vi "ADC_write_read.vi"(8 "Sync_cnt":bool=TRUE, 11 "ADC  in":bool[](array[boolean])) -> (1 "ADC FIFO SYNC":u16=65532 format="%016b", 2 "ADC in":u32[](array[numeric]), 3 "ADC out":u32[](array[numeric]))   [LabVIEW 2015]
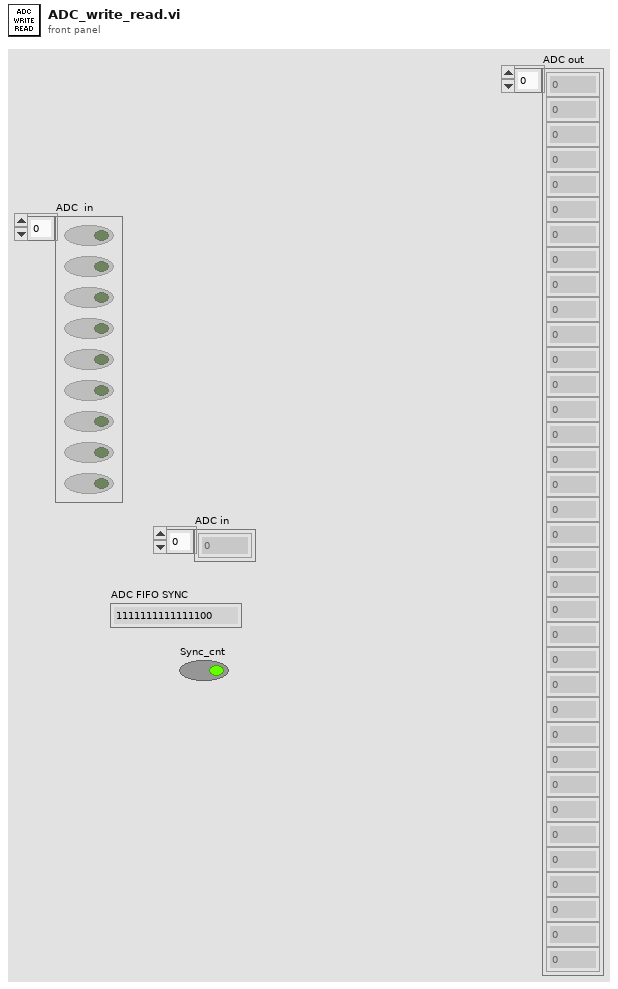
[diagram p1: front panel]
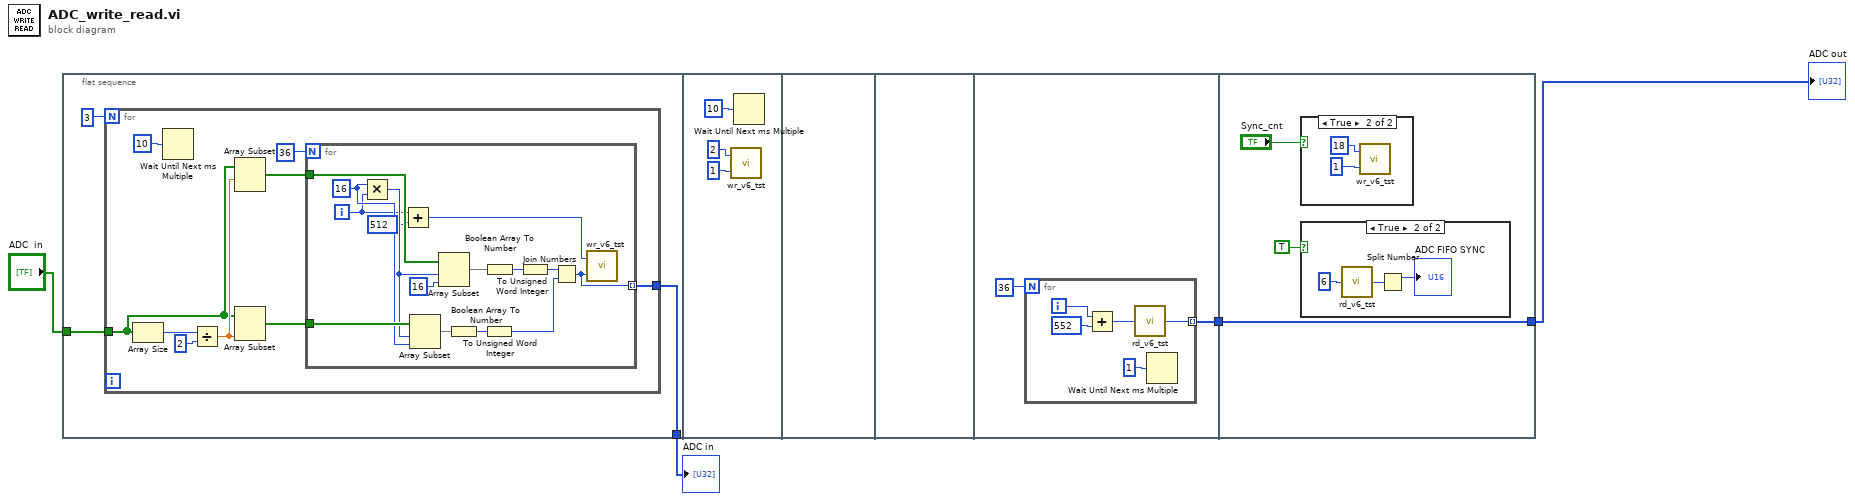
[diagram p0: block diagram]
diagram:
  n1 = flat-sequence {
    tunnel: "ADC  in" -> [w7]
    tunnel: [w6] -> w4
    tunnel: [w35] -> w2
    tunnel: [w44] -> w1
    tunnel: w2 -> [w44]
    frame #0 {
      n2 = for {
        N: 3 -> [_]
        tunnel: w7 -> [w10]
        tunnel: [w9] -> w6
        n3 = Array Size(array=w10) -> (size(s)=w11:i32)
        n4 = Wait Until Next ms Multiple(millisecond multiple=u32 10) -> ()  [unwired: 1 out]
        n5 = Divide(x=w11, y=2) -> (x/y=w16:dbl)
        n6 = Array Subset(array=w10, index=w16) -> (w14:bool[])  [unwired: 1 in]
        n7 = Array Subset(array=w10, length=w16) -> (w13:bool[])  [unwired: 1 in]
        n8 = for {
          N: 36 -> [_]
          tunnel: w13 -> [w31]
          tunnel: w14 -> [w29]
          tunnel: [w19] -> w9 mode=indexing
          i -> [w20]
          w30 = 16 ("length")
          n9 = Multiply(x=w30, y=w20) -> (x*y=w27:i32)
          n10 = Add(x=w20, y=512) -> (x+y=w18:i32)
          n11 = Array Subset(array=w31, index=w27, length=w30) -> (w23:bool[])
          n12 = Array Subset(array=w29, index=w27, length=16) -> (w24:bool[])
          n13 = Boolean Array To Number(Boolean array=w23) -> (number=w25:u32)
          n14 = To Unsigned Word Integer(number=w25) -> (unsigned 16bit integer=w22:u16)
          n15 = Boolean Array To Number(Boolean array=w24) -> (number=w26:u32)
          n16 = To Unsigned Word Integer(number=w26) -> (unsigned 16bit integer=w21:u16)
          n17 = Join Numbers(hi=w21, lo=w22) -> ((hi.lo)=w19:u32)
          n18 = call "wr_v6_tst.vi"("DATA"=w19, "ADDRESS"=w18) -> ()  [unwired: 1 out]
        }
      }
    }
    frame #1 {
      n19 = call "wr_v6_tst.vi"("DATA"=u32 1, "ADDRESS"=u16 2) -> ()  [unwired: 1 out]
      n20 = Wait Until Next ms Multiple(millisecond multiple=u32 10) -> ()  [unwired: 1 out]
    }
    frame #2 {
    }
    frame #3 {
    }
    frame #4 {
      n21 = for {
        N: 36 -> [_]
        tunnel: [w39] -> w35 mode=indexing
        i -> [w41]
        n22 = Add(x=w41, y=552) -> (x+y=w40:i32)
        n23 = call "rd_v6_tst.vi"("ADDRESS 2"=w40) -> ("DATA 2"=w39:u32)
        n24 = Wait Until Next ms Multiple(millisecond multiple=u32 1) -> ()  [unwired: 1 out]
      }
    }
    frame #5 {
      n25 = case shown="True" "Sync_cnt" {
        frame False {
        }
        frame True {
          n26 = call "wr_v6_tst.vi"("DATA"=u32 1, "ADDRESS"=u16 18) -> ()  [unwired: 1 out]
        }
      }
      n27 = case shown="True" TRUE {
        frame False {
        }
        frame True {
          n28 = call "rd_v6_tst.vi"("ADDRESS 2"=i16 6) -> ("DATA 2"=w48:u32)
          n29 = Split Number(x=w48) -> (hi(x)=→"ADC FIFO SYNC":u16)  [unwired: 1 out]
        }
      }
    }
  }
  "ADC out" <- w1
  "ADC in" <- w4
